vi "LVClass_DataClient GetInteger.vi"(0 "DataClient in":refnum<class "DataClient.lvclass">, 5 "name":string, 11 "error in (no error)":errorcluster) -> (4 "DataClient out":refnum<class "DataClient.lvclass">, 8 "Value":i32, 10 "data_unique_id":i32, 15 "error out":errorcluster)   [LabVIEW 2020, in "DataClient.lvclass"]
doc: "Slopes getter.\n\n<B>clientIn</B> : Client object.\n<B>clientOut</B> : Client object.\n<B>data_name</B> : Data name.\n<B>data</B> : Data content.\n<B>data_id</B> : Data content id."
uses:
  DataClient.lvclass
  DataClient.lvclass/DataClient.ctl
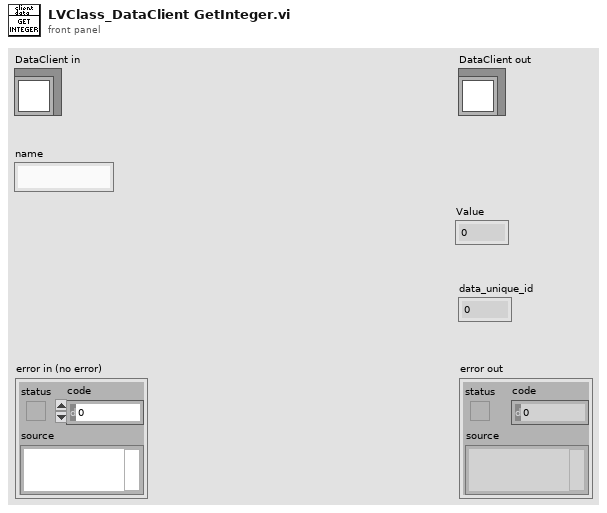
[diagram p1: front panel]
types:
  T1 = typedef "ClassID.ctl" = i64
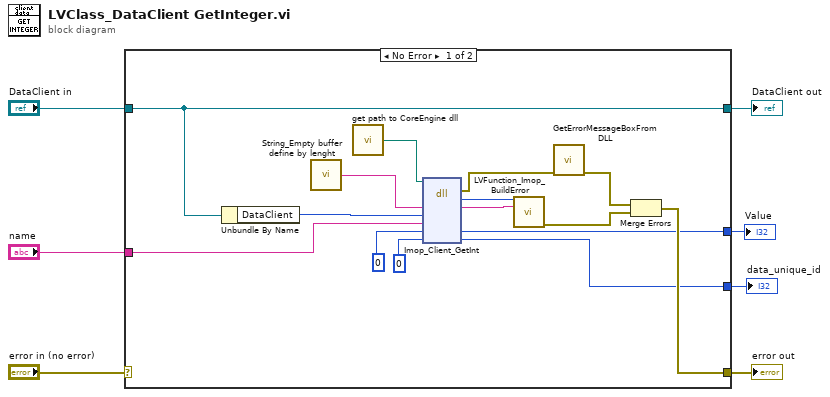
[diagram p0: block diagram]
diagram:
  n1 = case shown="No Error" "error in (no error)" {
    selector: "error in (no error)" -> [_ w24]
    tunnel: [w13 w24] -> w6
    tunnel: [w14 w23] -> w4
    tunnel: "DataClient in" -> [w14 w23]
    tunnel: "name" -> [w12 _]
    tunnel: [w10 _] -> w2
    tunnel: [w8 _] -> w1
    frame No Error {
      n2 = Unbundle By Name(w14) -> ("DataClient"=w17:T1)
      n3 = call "String_Empty buffer define by lenght.vi"() -> ("Empty buffer"=w20:string)  [unwired: 1 in]
      n4 = call "get path to CoreEngine dll.vi"() -> ("path to wavekit library"=w19:path)  [unwired: 14 in, 1 out]
      n5 = dll-call lib="D:/soft/HASO_v3/SVN_trunk/ImOpCoreEngine4_LV2011/DLLs/c_interface_vc100.dll" fn="Imop_Client_GetInt"(path in=w19, "message"=w20, "client"=w17, "name"=w12, "value"=0 ("bool"), "data_id"=0) -> (error out=w18:errorcluster, "return type"=w22:i32, "message"=w21:string, "value"=w8:i32, "data_id"=w10:i32)  [unwired: 4 in, 1 out]
      n6 = call "LVFunction_Imop_BuildError.vi"("code"=w22, "String to Prepend to source (\"\")"=w21) -> ("error out"=w15:errorcluster)  [unwired: 13 in]
      n7 = call "GetErrorMessageBoxFromDLL.vi"("error IN"=w18) -> ("error OUT"=w16:errorcluster)  [unwired: 10 in]
      n8 = Merge Errors(w16, w15) -> (w13:errorcluster)
    }
    frame Error {
    }
  }
  "error out" <- w6
  "DataClient out" <- w4
  "Value" <- w1
  "data_unique_id" <- w2
